vi "NumIntegrate_Rk4_Mat_X_U.vi"(5 "Func_X_U_Extra":T1, 7 "PassedData":variant, 8 "dT_Seconds":dbl, 10 "U":T2, 11 "X":T2) -> (0 "Error":bool, 3 "OUTPUT":T2)   [LabVIEW 2019, in "Trajectory_Library.lvlib"]
doc: "Performs 4th order Runge-Kutta integration of dx/dt = f( matrix x, matrix u) for dt.\n\nInputs:\n - Func_X_U_Extra -- A strictly typed LabVIEW reference to a function to integrate as a function of matrix X, U, and the extra passed data\n - PassedData -- This is a variant that can be used to pass additional data to the function if needed. The data must be packed into the variant in the specific way expected by the function.\n - X -- X input matrix\n - U -- U input matrix.\n - dT -- Time differential in seconds\n\nOutputs:\n - OUTPUT -- The integration of dx/dt = f(x, u) for dt.\n - Error -- If TRUE, an error occured."
uses:
  Trajectory_Library.lvlib
  <vilib>/Analysis/Matrix/Datatypes/RealMatrix.ctl
  CALLBACK_FUNC_TYPE.ctl
  <vilib>/Analysis/Matrix/Numeric/Multiply/Multiply - RM,R.vi
  <vilib>/Analysis/Matrix/Numeric/Add/Add - RM,RM.vi
  <vilib>/Analysis/Matrix/NI_Matrix.lvlib
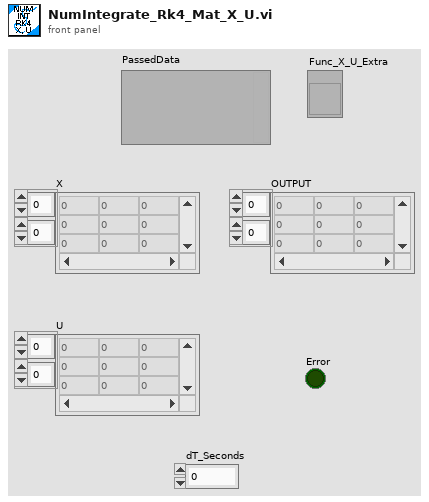
[diagram p1: front panel]
types:
  T1 = typedef "Trajectory_Library.lvlib/CALLBACK_FUNC_TYPE.ctl" = refnum<vi>
  T2 = typedef "NI_Matrix.lvlib/RealMatrix.ctl" = dbl[][]
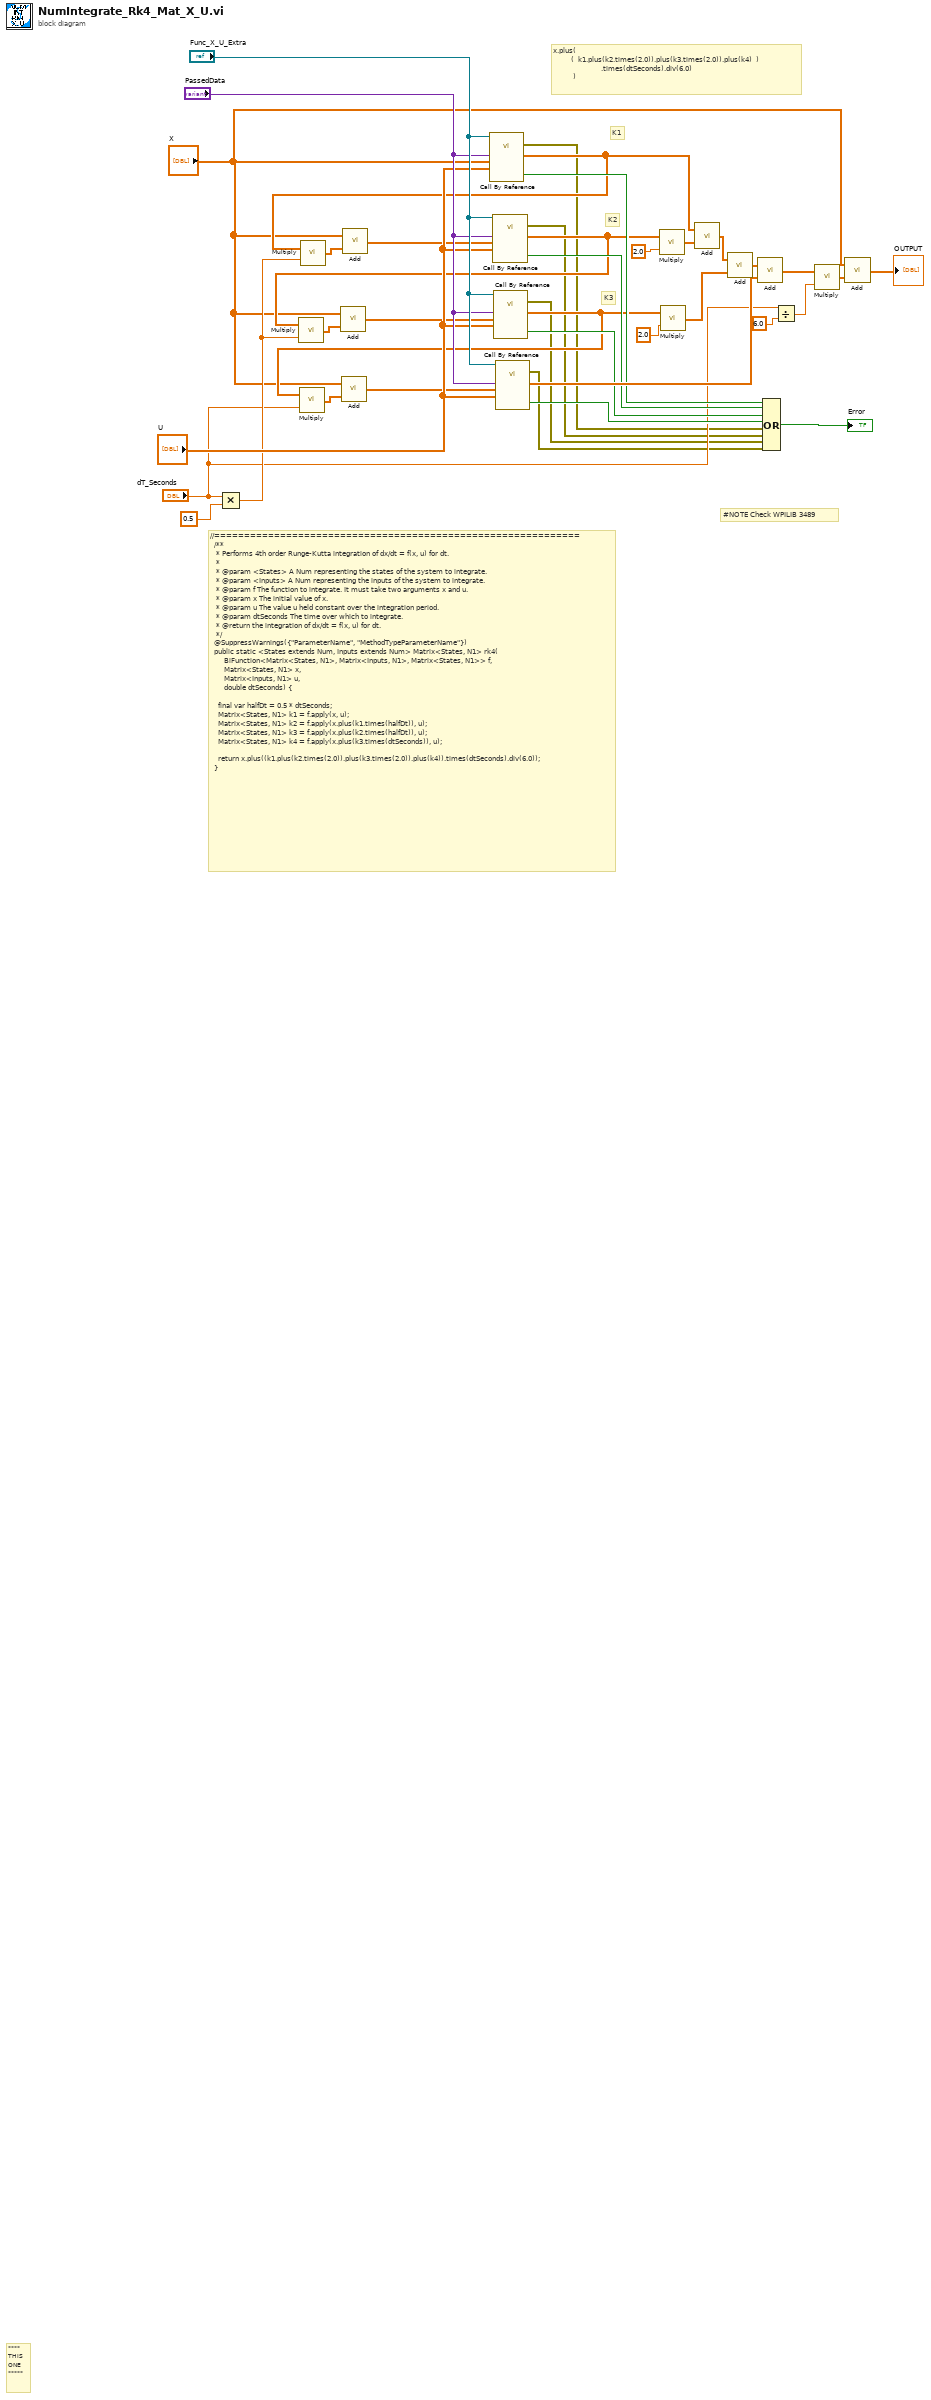
[diagram p0: block diagram]
diagram:
  # "#NOTE Check WPILIB 3489"
  # "x.plus(\n         (  k1.plus(k2.times(2.0)).plus(k3.times(2.0)).plus(k4)  )\n                        .times(dtSeconds).div(6.0)\n          )"
  # "K3"
  # "K2"
  # "K1"
  # "//=============================================================\n  /**\n   * Performs 4th order Runge-Kutta integration of dx/dt = f(x, u) for dt.\n   *\n   * @param <States> A Num representing the states of the system to integrate.\n   * @param <Inputs> A Num representing the inputs of the system to integrate.\n   * @param f The function to integrate. It must take two arguments x and u.\n   * @param x The initial value of x.\n   * @param u The value u held constant over the integration period.\n   * @param dtSeconds The time over which to integrate.\n   * @return the integration of dx/dt = f(x, u) for dt.\n   */\n  @SuppressWarnings({\"ParameterName\", \"MethodTypeParameterName\"})\n  public static <States extends Num, Inputs extends Num> Matrix<States, N1> rk4(\n      \tBiFunction<Matrix<States, N1>, Matrix<Inputs, N1>, Matrix<States, N1>> f,\n      \tMatrix<States, N1> x,\n      \tMatrix<Inputs, N1> u,\n      \tdouble dtSeconds) {\n\n    final var halfDt = 0.5 * dtSeconds;\n    Matrix<States, N1> k1 = f.apply(x, u);\n    Matrix<States, N1> k2 = f.apply(x.plus(k1.times(halfDt)), u);\n    Matrix<States, N1> k3 = f.apply(x.plus(k2.times(halfDt)), u);\n    Matrix<States, N1> k4 = f.apply(x.plus(k3.times(dtSeconds)), u);\n\n    return x.plus((k1.plus(k2.times(2.0)).plus(k3.times(2.0)).plus(k4)).times(dtSeconds).div(6.0));\n  }"
  # "****\nTHIS\nONE\n*****"
  n1 = Multiply(x="dT_Seconds", y=0.5) -> (x*y=w12:dbl)
  n2 = call-by-ref "?"(reference="Func_X_U_Extra", "U"="U", "X"="X", "Variant"="PassedData") -> (error out=w4:errorcluster, "Error"=w27:bool, "NewX"=w21:T2)  [unwired: 8 in, 1 out]
  n3 = call-poly <vilib>:"Multiply.vi"("Real Scalar c"=w12, "Real Matrix A"=w21) -> ("A * c"=w20:T2)
  n4 = call-poly <vilib>:"Add.vi"("Real Matrix B"=w20, "Real Matrix A"="X") -> ("A + B"=w19:T2)
  n5 = call-by-ref "?"(reference="Func_X_U_Extra", "U"="U", "X"=w19, "Variant"="PassedData") -> (error out=w3:errorcluster, "Error"=w26:bool, "NewX"=w16:T2)  [unwired: 8 in, 1 out]
  n6 = call-poly <vilib>:"Multiply.vi"("Real Scalar c"=w12, "Real Matrix A"=w16) -> ("A * c"=w18:T2)
  n7 = call-poly <vilib>:"Add.vi"("Real Matrix B"=w18, "Real Matrix A"="X") -> ("A + B"=w17:T2)
  n8 = call-by-ref "?"(reference="Func_X_U_Extra", "U"="U", "X"=w17, "Variant"="PassedData") -> (error out=w2:errorcluster, "Error"=w25:bool, "NewX"=w13:T2)  [unwired: 8 in, 1 out]
  n9 = call-poly <vilib>:"Multiply.vi"("Real Scalar c"="dT_Seconds", "Real Matrix A"=w13) -> ("A * c"=w15:T2)
  n10 = call-poly <vilib>:"Add.vi"("Real Matrix B"=w15, "Real Matrix A"="X") -> ("A + B"=w14:T2)
  n11 = call-by-ref "?"(reference="Func_X_U_Extra", "U"="U", "X"=w14, "Variant"="PassedData") -> (error out=w1:errorcluster, "Error"=w24:bool, "NewX"=w28:T2)  [unwired: 8 in, 1 out]
  n12 = call-poly <vilib>:"Multiply.vi"("Real Scalar c"=2.0, "Real Matrix A"=w16) -> ("A * c"=w32:T2)
  n13 = call-poly <vilib>:"Multiply.vi"("Real Scalar c"=2.0, "Real Matrix A"=w13) -> ("A * c"=w30:T2)
  n14 = call-poly <vilib>:"Add.vi"("Real Matrix B"=w32, "Real Matrix A"=w21) -> ("A + B"=w31:T2)
  n15 = call-poly <vilib>:"Add.vi"("Real Matrix B"=w30, "Real Matrix A"=w31) -> ("A + B"=w29:T2)
  n16 = call-poly <vilib>:"Add.vi"("Real Matrix B"=w28, "Real Matrix A"=w29) -> ("A + B"=w11:T2)
  n17 = Compound Arithmetic op=OR(w27, w26, w25, w24, w4, w3, w2, w1) -> (→"Error":bool)
  n18 = Divide(x="dT_Seconds", y=6.0) -> (x/y=w8:dbl)
  n19 = call-poly <vilib>:"Multiply.vi"("Real Scalar c"=w8, "Real Matrix A"=w11) -> ("A * c"=w7:T2)
  n20 = call-poly <vilib>:"Add.vi"("Real Matrix B"=w7, "Real Matrix A"="X") -> ("A + B"=→"OUTPUT":T2)
